vi "MicroZed Write.vi"(8 "Error In":errorcluster, 9 "PC Config":T1={"AC Voltage SP"=0.0, "AC Current SP"=0.0, "Frequency SP"=60.0, "DC Voltage SP"=0.0, "Op Mode SP"=enum."Shutdown (Reset)", "Clear Faults SP"=0} {"Clear Faults SP" format="%01x"; "DC Voltage SP" min=300 max=550 format="%2.1f"; "Frequency SP" min=45 max=65 format="%2.1f"; "AC Current SP" min=-500 max=500 format="%2.1f"; "AC Voltage SP" min=0 max=132 format="%2.1f"}, 11 "TCP Master Ref In":refnum<class "Modbus Master.lvclass">) -> (0 "Error Out":errorcluster, 3 "TCP Master Ref Out":refnum<class "Modbus Master.lvclass">)   [LabVIEW 2014]
uses:
  <vilib>/Modbus/master/Modbus Master.lvclass
  Controls/MicroZed Config.ctl
  Controls/MicroZed Config Op Mode.ctl
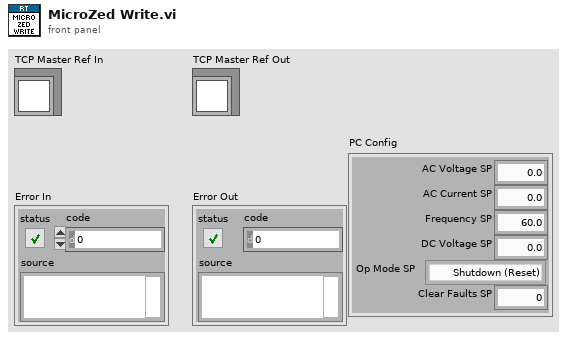
[diagram p1: front panel]
types:
  T1 = typedef "MicroZed Config.ctl" = cluster{"AC Voltage SP":sgl, "AC Current SP":sgl, "Frequency SP":sgl, "DC Voltage SP":sgl, "Op Mode SP":T2, "Clear Faults SP":i16}
  T2 = typedef "MicroZed Config Op Mode.ctl" = enum16{"Shutdown (Reset)", "Startup", "Idle", "Voltage Mode", "Current Mode", "Fault", "OL Voltage (Debug)", "No Data"}
  T3 = cluster{"AC Voltage SP":bool, "AC Current SP":bool, "Frequency SP":bool, "DC Voltage SP":bool, "Op Mode SP":bool, "Clear Faults SP":bool}
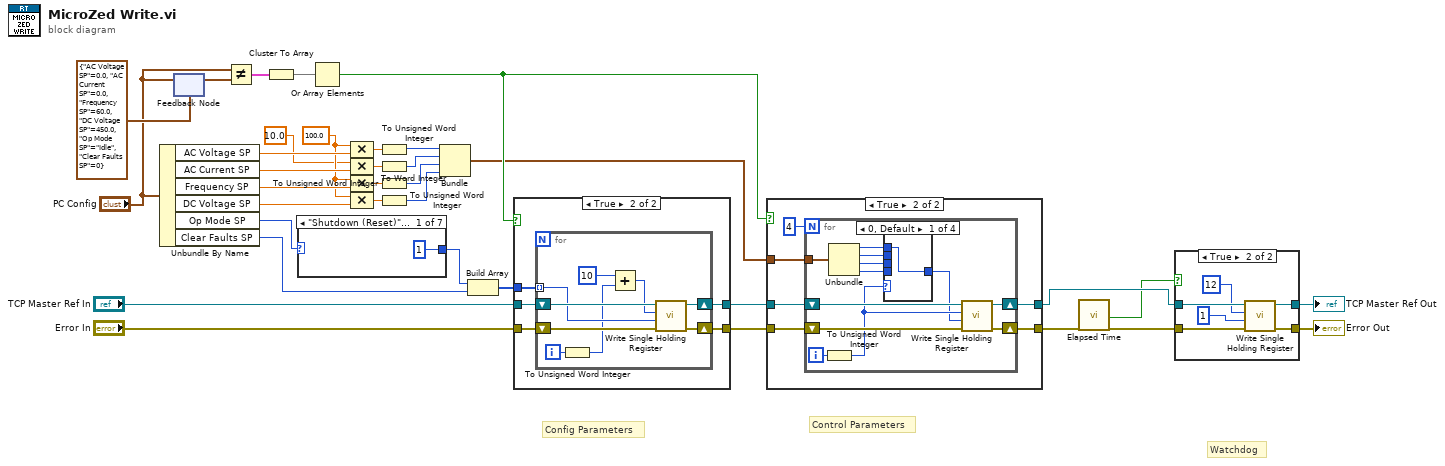
[diagram p0: block diagram]
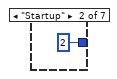
[diagram p3: hidden frame]
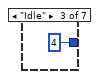
[diagram p4: hidden frame]
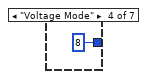
[diagram p5: hidden frame]
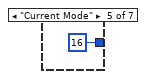
[diagram p6: hidden frame]
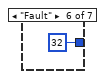
[diagram p7: hidden frame]
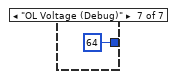
[diagram p8: hidden frame]
diagram:
  w22 = sgl 100.0
  # "Watchdog"
  # "Control Parameters"
  # "Config Parameters"
  n1 = Unbundle By Name("PC Config") -> ("AC Voltage SP"=w23:sgl, "AC Current SP"=w24:sgl, "Frequency SP"=w25:sgl, "DC Voltage SP"=w26:sgl, "Op Mode SP"=w19:T2, "Clear Faults SP"=w20:i16)
  n2 = feedback-in #1("PC Config") -> ()
  n3 = feedback #1(T1 {"AC Voltage SP"=0.0, "AC Current SP"=0.0, "Frequency SP"=60.0, "DC Voltage SP"=450.0, "Op Mode SP"=enum."Idle", "Clear Faults SP"=0} ("PC Config")) -> (w8:T1)
  n4 = Not Equal?(x="PC Config", y=w8) -> (x != y?=w33:T3)
  n5 = Cluster To Array(cluster=w33) -> (array=w32:bool[])
  n6 = case shown="\"Shutdown (Reset)\", Default" w19 {
    tunnel: [u16 1 u16 2 u16 4 u16 8 u16 16 u16 32 u16 64] -> w18
    frame "Shutdown (Reset)", Default {
    }
    frame "Startup" {
    }
    frame "Idle" {
    }
    frame "Voltage Mode" {
    }
    frame "Current Mode" {
    }
    frame "Fault" {
    }
    frame "OL Voltage (Debug)" {
    }
  }
  n7 = Or Array Elements(Boolean array=w32) -> (logical OR=w34:bool)
  n8 = Compound Arithmetic op=MULTIPLY(w22, w23) -> (w17:sgl)
  n9 = Compound Arithmetic op=MULTIPLY(sgl 10.0, w24) -> (w16:sgl)
  n10 = Compound Arithmetic op=MULTIPLY(w22, w25) -> (w15:sgl)
  n11 = Compound Arithmetic op=MULTIPLY(w22, w26) -> (w14:sgl)
  n12 = To Unsigned Word Integer(number=w17) -> (unsigned 16bit integer=w13:u16)
  n13 = To Word Integer(number=w16) -> (16bit integer=w12:i16)
  n14 = To Unsigned Word Integer(number=w15) -> (unsigned 16bit integer=w11:u16)
  n15 = To Unsigned Word Integer(number=w14) -> (unsigned 16bit integer=w10:u16)
  n16 = Bundle(w13, w12, w11, w10) -> (w9:cluster{u16, i16, u16, u16})  [unwired: 1 in]
  n17 = Build Array(w18, w20) -> (w31:u16[])
  n18 = case shown="True" w34 {
    tunnel: "Error In" -> [w43 w49]
    tunnel: [w43 w48] -> w28
    tunnel: [w44 w47] -> w27
    tunnel: "TCP Master Ref In" -> [w44 w46]
    tunnel: w31 -> [_ w45]
    frame False {
    }
    frame True {
      n19 = for {
        shift-right: [w57] -> w48
        shift-left: w49 -> [w58]
        shift-right: [w56] -> w47
        shift-left: w46 -> [w55]
        tunnel: w45 -> [w53] mode=indexing
        i -> [w51]
        n20 = To Unsigned Word Integer(number=w51) -> (unsigned 16bit integer=w50:u16)
        n21 = Add(x=u16 10 ("starting address"), y=w50) -> (x+y=w52:u16)
        n22 = call-dynamic "Write Single Holding Register.vi"("error in (no error)"=w58, "holding register value"=w53, "address"=w52, "Modbus master in"=w55) -> ("error out"=w57:errorcluster, "Modbus master out"=w56:refnum<class "Modbus Master.lvclass">)  [unwired: 6 in]
      }
    }
  }
  n23 = case shown="True" w34 {
    tunnel: w28 -> [w59 w66]
    tunnel: w27 -> [w60 w65]
    tunnel: [w59 w64] -> w4
    tunnel: [w60 w63] -> w2
    tunnel: w9 -> [_ w62]
    frame False {
    }
    frame True {
      n24 = for {
        N: 4 -> [_]
        shift-right: [w76] -> w64
        shift-left: w66 -> [w78]
        shift-right: [w75] -> w63
        shift-left: w65 -> [w77]
        tunnel: w62 -> [w72]
        i -> [w74]
        n25 = To Unsigned Word Integer(number=w74) -> (unsigned 16bit integer=w73:u16)
        n26 = Unbundle(w72) -> (w71:u16, w70:i16, w69:u16, w68:u16)
        n27 = case shown="0, Default" w73 {
          tunnel: w71 -> [w79 _ _ _]
          tunnel: w70 -> [_ w80 _ _]
          tunnel: w69 -> [_ _ w81 _]
          tunnel: w68 -> [_ _ _ w82]
          tunnel: [w79 w80 w81 w82] -> w67
          frame 0, Default {
          }
          frame 1 {
          }
          frame 2 {
          }
          frame 3 {
          }
        }
        n28 = call-dynamic "Write Single Holding Register.vi"("error in (no error)"=w78, "holding register value"=w67, "address"=w73, "Modbus master in"=w77) -> ("error out"=w76:errorcluster, "Modbus master out"=w75:refnum<class "Modbus Master.lvclass">)  [unwired: 6 in]
      }
    }
  }
  n29 = call "Elapsed Time"("error in (no error)"=w4) -> ("Time has Elapsed"=w1:bool, "error out"=w3:errorcluster)  [unwired: 11 in, 6 out]
  n30 = case shown="True" w1 {
    tunnel: w3 -> [w84 w90]
    tunnel: [w84 w89] -> w6
    tunnel: w2 -> [w83 w88]
    tunnel: [w83 w87] -> w5
    frame False {
    }
    frame True {
      n31 = call-dynamic "Write Single Holding Register.vi"("error in (no error)"=w90, "holding register value"=u16 1, "address"=u16 12, "Modbus master in"=w88) -> ("error out"=w89:errorcluster, "Modbus master out"=w87:refnum<class "Modbus Master.lvclass">)  [unwired: 6 in]
    }
  }
  "Error Out" <- w6
  "TCP Master Ref Out" <- w5
